vi "Read Sub Panel Monedas.vi"(8 "error in (no error)":errorcluster, 11 "Quetzal Actor in":refnum<class "Quetzal Actor.lvclass">) -> (0 "error out":errorcluster, 2 "Sub Panel Monedas":refnum<vi>, 3 "Quetzal Actor out":refnum<class "Quetzal Actor.lvclass">)   [LabVIEW 2020, in "Quetzal Actor.lvlib" / "Quetzal Actor.lvclass"]
uses:
  Quetzal Actor.lvclass
  Quetzal Actor.lvclass/Quetzal Actor.ctl
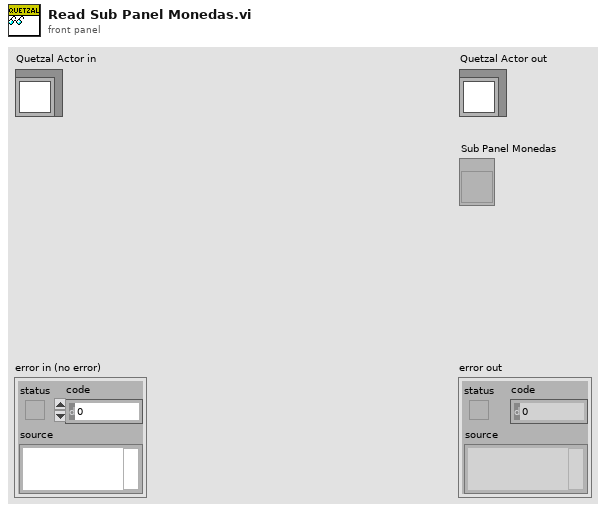
[diagram p1: front panel]
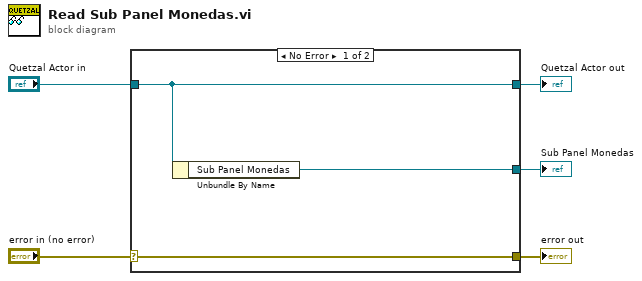
[diagram p0: block diagram]
diagram:
  n1 = case shown="No Error" "error in (no error)" {
    selector: "error in (no error)" -> [w8 w9]
    tunnel: [w8 w9] -> w4
    tunnel: [w7 w10] -> w2
    tunnel: "Quetzal Actor in" -> [w7 w10]
    tunnel: [w6 _] -> w1
    frame No Error {
      n2 = Unbundle By Name(w7) -> ("Sub Panel Monedas"=w6:refnum<vi>)
    }
    frame Error {
    }
  }
  "error out" <- w4
  "Quetzal Actor out" <- w2
  "Sub Panel Monedas" <- w1
